vi "test_inline_table_write_key_string.vi"(8 "error in (no error)":errorcluster) -> (0 "error out":errorcluster)   [LabVIEW 2020]
uses:
  f3be1312-b272-4eb0-9337-bd000e73fd02.vi
  f3be1312-b272-4eb0-9337-bd000e73fd02.vi/4178f046-9af6-4db4-9405-99552d650b27.vi
  f3be1312-b272-4eb0-9337-bd000e73fd02.vi/504846f3-46c1-483c-ab2c-e4b1da560c38.vi
  toml/write_subtable_key_string.vi
  toml/toml.lvclass
  <vilib>/addons/_JKI Toolkits/Caraya/classes/Assert/Assert.lvclass
  <vilib>/addons/_JKI Toolkits/Caraya/classes/Test/Test.lvclass
panel:
  out "toml_string":string
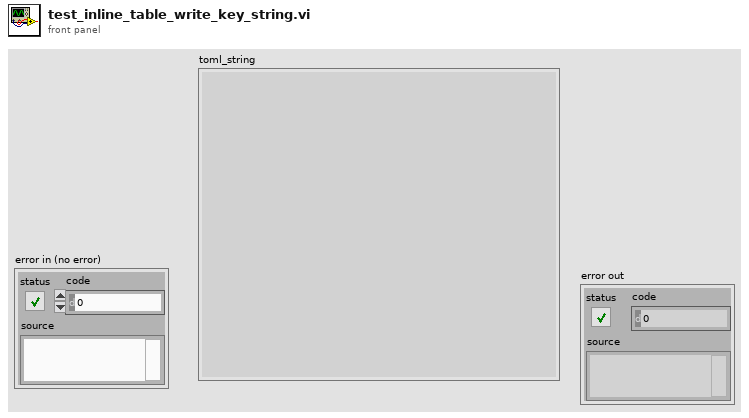
[diagram p1: front panel]
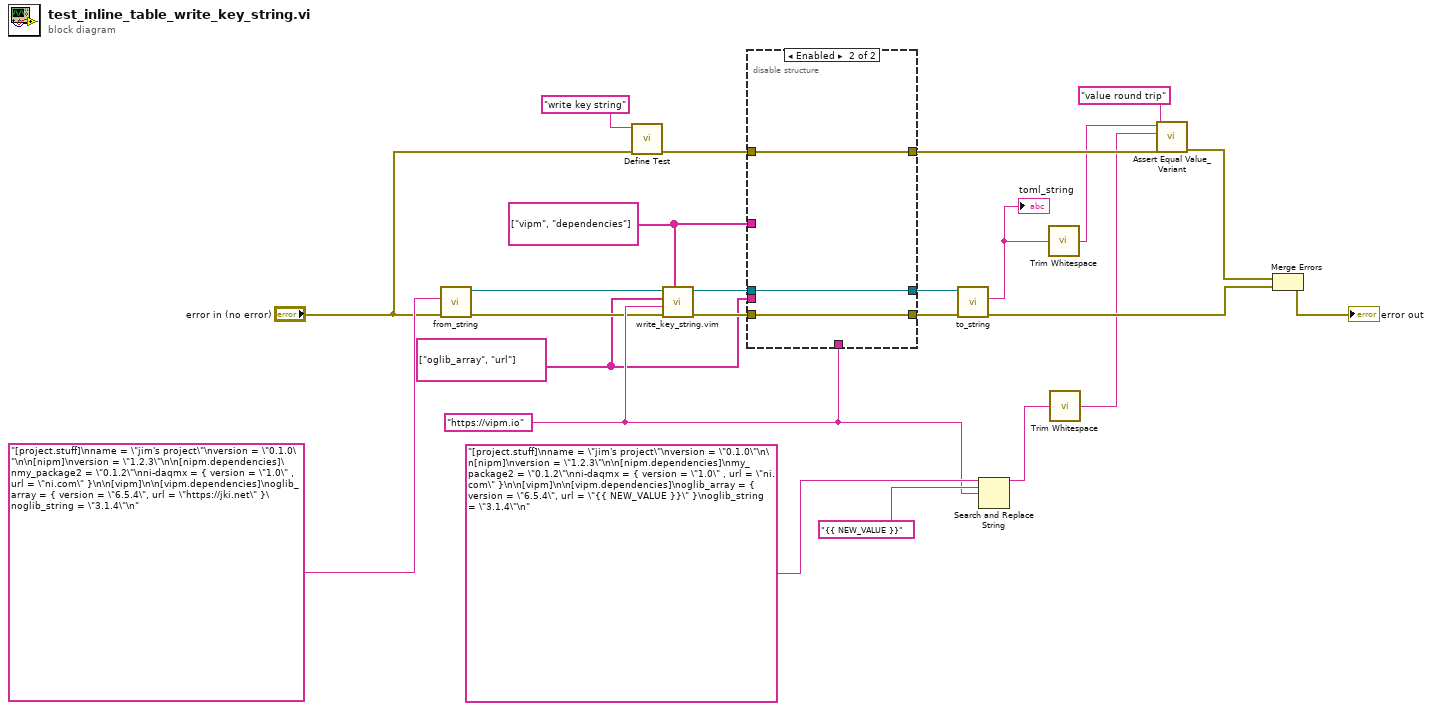
[diagram p0: block diagram]
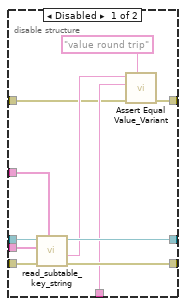
[diagram p2: hidden frame]
diagram:
  w2 = string[] ["oglib_array", "url"]
  w3 = string[] ["vipm", "dependencies"]
  w5 = "https://vipm.io" ("string")
  n1 = call "from_string.vi"("error in (no error)"="error in (no error)", "toml"="[project.stuff]\nname = \"jim's project\"\nversion = \"0.1.0\"\n\n[nipm]\nversion = \"1.2.3\"\n\n[nipm.dependencies]\nmy_package2 = \"0.1.2\"\nni-daqmx = { version = \"1.0\" , url = \"ni.com\" }\n\n[vipm]\n\n[vipm.dependencies]\noglib_array = { version = \"6.5.4\", url = \"https://jki.net\" }\noglib_string = \"3.1.4\"\n" ("toml_string in")) -> ("error out"=w4:errorcluster, "toml out"=w6:refnum<class "toml.lvclass">)  [unwired: 8 in]
  n2 = call <vilib>:"Define Test.vi"("error in (no error)"="error in (no error)", "Label (VI Title)"="write key string") -> ("error out"=w11:errorcluster)  [unwired: 9 in]
  n3 = call "write_key_string.vim"("table"=w3, "error in (no error)"=w4, "value"=w5, "key"=w2, "toml in"=w6) -> ("error out"=w23:errorcluster, "toml out"=w21:refnum<class "toml.lvclass">)  [unwired: 5 in]
  n4 = disable-structure shown="Enabled" {
    disable-tunnel: w23 -> [w35 w36]
    disable-tunnel: [w34 w36] -> w22
    disable-tunnel: w21 -> [w33 w37]
    disable-tunnel: [w32 w37] -> w20
    disable-tunnel: w3 -> [w25 _]
    disable-tunnel: w2 -> [w31 _]
    disable-tunnel: [w29 w38] -> w19
    disable-tunnel: w5 -> [w27 _]
    disable-tunnel: w11 -> [w26 w38]
    frame Disabled {
      n5 = call "read_subtable_key_string.vi"("subtables"=w25, "error in (no error)"=w35, "key"=w31, "toml in"=w33) -> ("error out"=w34:errorcluster, "value"=w30:string, "toml out"=w32:refnum<class "toml.lvclass">)  [unwired: 5 in]
      n6 = call <vilib>:"Assert Equal Value_Variant.vi"("Label"="value round trip", "error in (no error)"=w26, "Y"=w27, "X"=w30) -> ("error out"=w29:errorcluster)  [unwired: 7 in]
    }
    frame Enabled {
    }
  }
  n7 = call "to_string.vi"("error in (no error)"=w22, "toml in"=w20) -> ("error out"=w16:errorcluster, "toml_string"=w9:string)  [unwired: 8 in]
  "toml_string" <- w9
  n8 = Search and Replace String(input string="[project.stuff]\nname = \"jim's project\"\nversion = \"0.1.0\"\n\n[nipm]\nversion = \"1.2.3\"\n\n[nipm.dependencies]\nmy_package2 = \"0.1.2\"\nni-daqmx = { version = \"1.0\" , url = \"ni.com\" }\n\n[vipm]\n\n[vipm.dependencies]\noglib_array = { version = \"6.5.4\", url = \"{{ NEW_VALUE }}\" }\noglib_string = \"3.1.4\"\n" ("toml_string in"), search string="{{ NEW_VALUE }}", replace string=w5) -> (result string=w1:string)  [unwired: 5 in, 3 out]
  n9 = call <vilib>:"Trim Whitespace.vi"("string"=w9) -> ("trimmed string"=w8:string)  [unwired: 1 in]
  n10 = call <vilib>:"Trim Whitespace.vi"("string"=w1) -> ("trimmed string"=w7:string)  [unwired: 1 in]
  n11 = call <vilib>:"Assert Equal Value_Variant.vi"("Label"="value round trip", "error in (no error)"=w19, "Y"=w7, "X"=w8) -> ("error out"=w17:errorcluster)  [unwired: 7 in]
  n12 = Merge Errors(w17, w16) -> (→"error out":errorcluster)
